vi "BML Write Pattern TEST.vi"() -> ()   [LabVIEW 2016]
uses:
  Classes/Config_Read/Config_Read.lvclass
  Classes/BML_Write/BML_Write.lvclass
  C:/Users/Zijun/Desktop/zijun_PXI_dev/Solutions/5g_eap/trunk/1.0/HiSi5GmmWave/BeamLink/BML_Pattern_Gen/Classes/BML_Root/BML_Root.lvclass
  Classes/BML_Root/BML_Root.lvclass/BML_Root.ctl
  Classes/BML_Write_Read/BML_Write_Read.lvclass
  Classes/BML_Root/BML_Root.lvclass
panel:
  out "error out":errorcluster
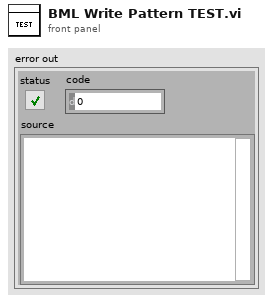
[diagram p1: front panel]
types:
  T1 = typedef "Config_Read.lvclass/Frame_Data.ctl" = cluster{"Pattern_Name":string, "Operation Mode":T2, "BurstLength":T3, "FSN":u8, "Start_Addr":u16, "Data":u8[], "R/W?":T4}
  T2 = typedef "Config_Read.lvclass/OperationMode.ctl" = enum8{"Normal", "ImmeEffect", "InitSlaveID", "LoadData"}
  T3 = typedef "Config_Read.lvclass/BurstLength.ctl" = enum8{"0", "2", "3", "4", "5", "8", "16", "32"}
  T4 = typedef "Config_Read.lvclass/RW_Option.ctl" = enum16{"Read", "Write", "R/W"}
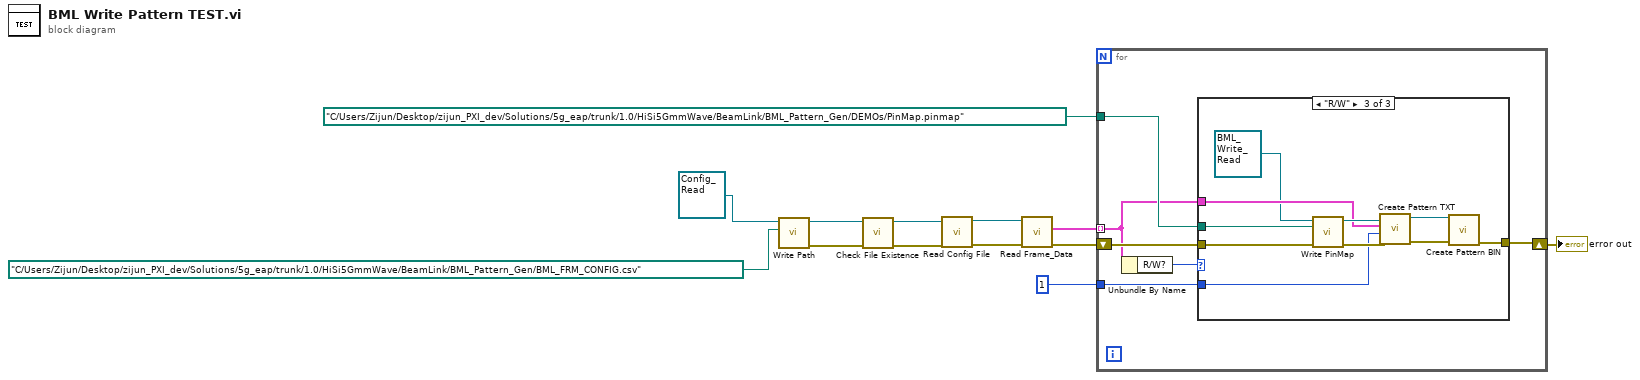
[diagram p0: block diagram]
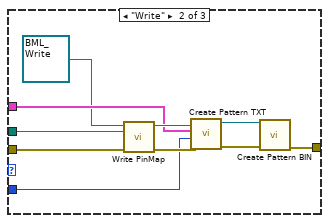
[diagram p3: hidden frame]
diagram:
  n1 = call-dynamic "Write Path.vi"("Path"=path "C:/Users/Zijun/Desktop/zijun_PXI_dev/Solutions/5g_eap/trunk/1.0/HiSi5GmmWave/BeamLink/BML_Pattern_Gen/BML_FRM_CONFIG.csv", "Config_Read in"=refnum<class "Config_Read.lvclass"> refnum ("Config_Read.lvclass")) -> ("error out"=w10:errorcluster, "Config_Read out"=w11:refnum<class "Config_Read.lvclass">)  [unwired: 8 in]
  n2 = call-dynamic "Check File Existence.vi"("error in (no error)"=w10, "Config_Read in"=w11) -> ("error out"=w8:errorcluster, "Config_Read out"=w9:refnum<class "Config_Read.lvclass">)  [unwired: 8 in]
  n3 = call-dynamic "Read Config File.vi"("error in (no error)"=w8, "Config_Read in"=w9) -> ("error out"=w6:errorcluster, "Config_Read out"=w7:refnum<class "Config_Read.lvclass">)  [unwired: 8 in]
  n4 = call-dynamic "Read Frame_Data.vi"("error in (no error)"=w6, "Config_Read in"=w7) -> ("error out"=w4:errorcluster, "FRM_Data_Array"=w5:T1[])  [unwired: 7 in, 1 out]
  n5 = for {
    tunnel: w5 -> [w16] mode=indexing
    shift-right: [w14] -> w1
    shift-left: w4 -> [w18]
    tunnel: path "C:/Users/Zijun/Desktop/zijun_PXI_dev/Solutions/5g_eap/trunk/1.0/HiSi5GmmWave/BeamLink/BML_Pattern_Gen/DEMOs/PinMap.pinmap" ("PinMap") -> [w19]
    tunnel: u8 1 ("ChipID") -> [w17]
    n6 = Unbundle By Name(w16) -> ("R/W?"=w15:T4)
    n7 = case shown="\"R/W\"" w15 {
      tunnel: w19 -> [_ w28 w38]
      tunnel: w18 -> [w20 w22 w32]
      tunnel: w17 -> [_ w27 w37]
      tunnel: w16 -> [_ w26 w36]
      tunnel: [w20 w23 w33] -> w14
      frame "Read", Default {
      }
      frame "Write" {
        n8 = call "Write PinMap.vi"("error in (no error)"=w22, "PinMap"=w28, "BML_Root in"=refnum<class "BML_Write.lvclass"> refnum ("BML_Write.lvclass")) -> ("error out"=w30:errorcluster, "BML_Root out"=w29:refnum<class "BML_Write.lvclass">)  [unwired: 7 in]
        n9 = call-dynamic "Create Pattern TXT.vi"("error in (no error)"=w30, "ChipID"=w27, "Frame_Data"=w26, "BML_Write in"=w29) -> ("error out"=w25:errorcluster, "BML_Write out"=w24:refnum<class "BML_Write.lvclass">)  [unwired: 6 in]
        n10 = call "Create Pattern BIN.vi"("error in (no error)"=w25, "BML_Root in"=w24) -> ("error out"=w23:errorcluster)  [unwired: 8 in, 1 out]
      }
      frame "R/W" {
        n11 = call "Write PinMap.vi"("error in (no error)"=w32, "PinMap"=w38, "BML_Root in"=refnum<class "BML_Write_Read.lvclass"> refnum ("BML_Write_Read.lvclass")) -> ("error out"=w40:errorcluster, "BML_Root out"=w39:refnum<class "BML_Write_Read.lvclass">)  [unwired: 7 in]
        n12 = call-dynamic "Create Pattern TXT.vi"("error in (no error)"=w40, "ChipID"=w37, "Frame_Data"=w36, "BML_Write_Read in"=w39) -> ("error out"=w35:errorcluster, "BML_Write_Read out"=w34:refnum<class "BML_Write_Read.lvclass">)  [unwired: 6 in]
        n13 = call "Create Pattern BIN.vi"("error in (no error)"=w35, "BML_Root in"=w34) -> ("error out"=w33:errorcluster)  [unwired: 8 in, 1 out]
      }
    }
  }
  "error out" <- w1
